vi "gl_Subpanel VI ref.vi"() -> ()   [LabVIEW 2020]
panel:
  out "Subpanel VI ref":refnum<vi>
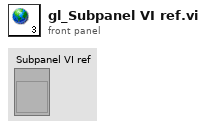
[diagram p1: front panel]
diagram:
